vi "Read File.vi"(7 "Address":string, 8 "Error In":errorcluster) -> (0 "Error Out":errorcluster)   [LabVIEW 2018, in "Tests.lvlib" / "KnownHosts.lvlib"]
uses:
  KnownHosts.lvlib
  <vilib>/Utility/error.llb/Clear Errors.vi
  <vilib>/Utility/file.llb/Is Path and Not Empty.vi
  <vilib>/Utility/sysdir.llb/Get System Directory.vi
  <vilib>/addons/_JKI Toolkits/Caraya/classes/Test/Test.lvclass
  <vilib>/addons/_JKI Toolkits/Caraya/classes/Assert/Assert.lvclass
  src/Toolkit/API/KnownHosts/Known Hosts.lvclass
  Tests.lvlib
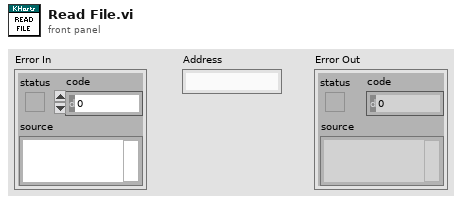
[diagram p1: front panel]
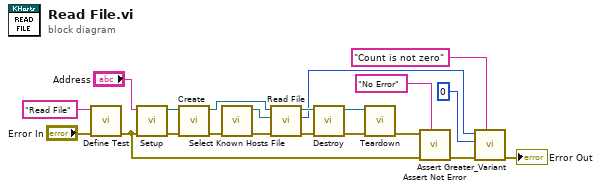
[diagram p0: block diagram]
diagram:
  n1 = call <vilib>:"Define Test.vi"("error in (no error)"="Error In", "Label (VI Title)"="Read File") -> ("error out"=w2:errorcluster)  [unwired: 9 in]
  n2 = call "Setup.vi"("Error In"=w2, "Address In"="Address") -> ("Error Out"=w5:errorcluster, "Sesssion"=w4:refnum<class "Session.lvclass">)  [unwired: 7 in, 1 out]
  n3 = call "Create.vi"("Error In"=w5, "Session"=w4) -> ("Error Out"=w10:errorcluster, "Known Hosts"=w17:refnum<class "Known Hosts.lvclass">)  [unwired: 8 in]
  n4 = call "Select Known Hosts File.vi"("Error In"=w10) -> ("Error Out"=w9:errorcluster, "Known Hosts File"=w8:path)  [unwired: 9 in]
  n5 = call "Read File.vi"("Error In"=w9, "File"=w8, "KnownHosts In"=w17) -> ("Error Out"=w16:errorcluster, "Count"=w13:u64, "KnownHosts Out"=w15:refnum<class "Known Hosts.lvclass">)  [unwired: 6 in]
  n6 = call "Destroy.vi"("Error In"=w16, "KnownHosts"=w15) -> ("Error Out"=w7:errorcluster, "Session"=w1:refnum<class "Session.lvclass">)  [unwired: 8 in]
  n7 = call "Teardown.vi"("Error In"=w7, "Session"=w1) -> ("Error Out"=w6:errorcluster)  [unwired: 9 in]
  n8 = call <vilib>:"Assert Not Error.vi"("Label"="No Error", "error in (no error)"=w2, "Not Error?"=w6) -> ("error out"=w18:errorcluster)  [unwired: 8 in]
  n9 = call <vilib>:"Assert Greater_Variant.vi"("Label"="Count is not zero", "error in (no error)"=w18, "Y"=u64 0 ("Count"), "X"=w13) -> ("error out"=→"Error Out":errorcluster)  [unwired: 7 in]
